vi "hasAttributeByType.vi"(7 "Attribute Type":refnum<class "Attribute.lvclass">, 8 "error in (no error)":errorcluster, 11 "SMO in":refnum<class "SMO.lvclass">) -> (0 "error out":errorcluster, 1 "found":bool, 3 "SMO out":refnum<class "SMO.lvclass">)   [LabVIEW 2013, in "SMO.lvclass"]
uses:
  SMO.lvclass
  Support/Attribute/Attribute.lvclass
  Support/Attribute/Attribute.lvclass/Attribute.ctl
  SMO.lvclass/SMO.ctl
  Private/ReftoDVR--SMO.vi
  <vilib>/Utility/LVClass/Get LV Class Name.vi
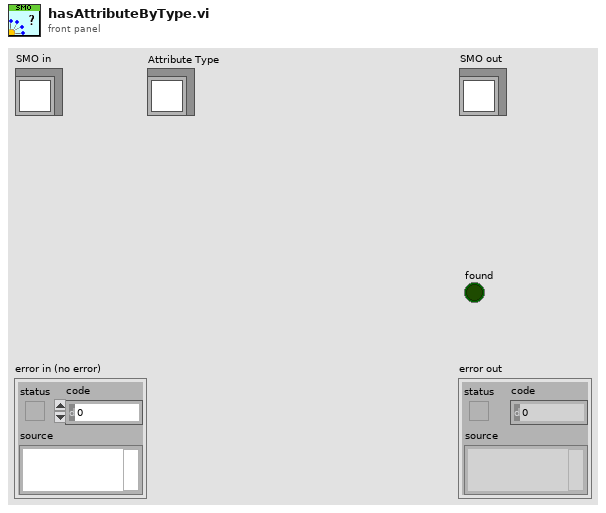
[diagram p1: front panel]
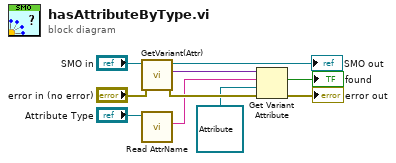
[diagram p0: block diagram]
diagram:
  n1 = call "GetVariant(Attr).vi"("error in (no error)"="error in (no error)", "SMO in"="SMO in") -> ("error out"=w8:errorcluster, "[Attributes]"=w6:variant, "SMO out"=→"SMO out":refnum<class "SMO.lvclass">)  [unwired: 7 in]
  n2 = call "Read AttrName.vi"("Attribute in"="Attribute Type") -> ("Attribute Name"=w3:string)  [unwired: 9 in, 1 out]
  n3 = Get Variant Attribute(Variant=w6, name=w3, default value (empty Variant)=refnum<class "Attribute.lvclass"> refnum ("Attribute.lvclass"), error in=w8) -> (found=→"found":bool, error out=→"error out":errorcluster)  [unwired: 2 out]
